vi "Get Picture.vi"(8 "error in (no error)":errorcluster, 11 "LED Array in":refnum<class "LED Array.lvclass">) -> (0 "error out":errorcluster, 2 "Picture":picture, 3 "LED Array out":refnum<class "LED Array.lvclass">)   [LabVIEW 2020, in "LED Array.lvclass"]
uses:
  LED Array.lvclass
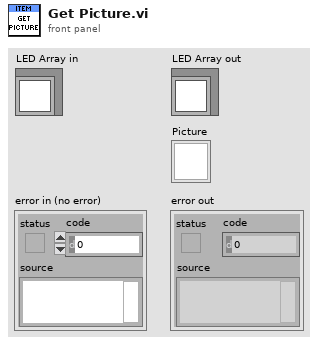
[diagram p1: front panel]
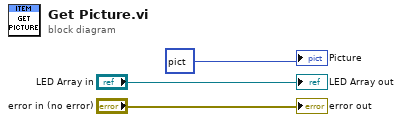
[diagram p0: block diagram]
diagram:
  "error out" <- "error in (no error)"
  "LED Array out" <- "LED Array in"
  "Picture" <- picture bytes[3230] ("new picture")
